vi "New Client.vi"(8 "error in (no error)":errorcluster, 9 "timeout ms (5000)":i32=5000, 11 "WebSocket URL":string) -> (0 "error out":errorcluster, 3 "WebSocket Client out":refnum<class "WebSocket Client.lvclass">)   [LabVIEW 2013, in "WebSockets.lvlib" / "WebSocket Client.lvclass"]
doc: "Opens a conenction and creates a new WebSocket Client using the NI VISA TCP Socket."
uses:
  WebSocket Client.lvclass
  WebSocket/WebSocket.lvclass/WebSocket.ctl
  WebSocket Client.lvclass/WebSocket Client.ctl
  WebSocket/Write Socket.vi
  Write URL.vi
  Sockets/VISA TCP Socket/VISA TCP.lvclass
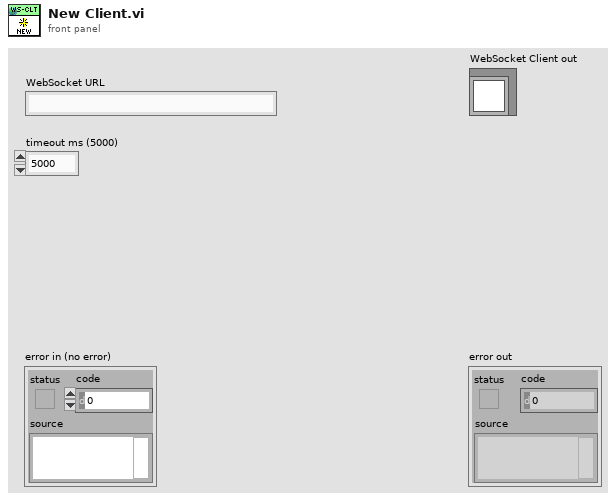
[diagram p1: front panel]
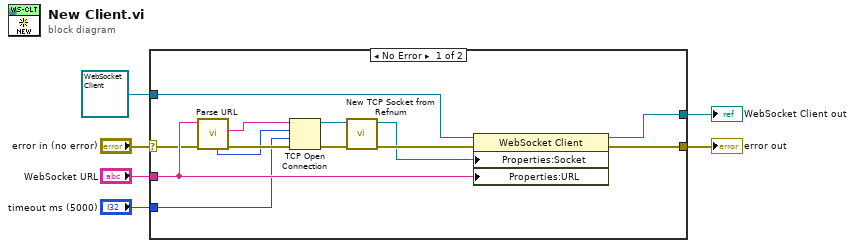
[diagram p0: block diagram]
diagram:
  n1 = case shown="No Error" "error in (no error)" {
    selector: "error in (no error)" -> [w7 w21]
    tunnel: refnum<class "WebSocket Client.lvclass"> refnum ("WebSocket Client in") -> [w19 w20]
    tunnel: [w18 w20] -> w5
    tunnel: [w17 w21] -> w4
    tunnel: "WebSocket URL" -> [w16 _]
    tunnel: "timeout ms (5000)" -> [w9 _]
    frame No Error {
      n2 = call "Parse URL.vi"("error in (no error)"=w7, "WebSocket URL"=w16) -> ("error out"=w10:errorcluster, "host"=w15:string, "port"=w8:u16)  [unwired: 5 in, 2 out]
      n3 = TCP Open Connection(address=w15, remote port or service name=w8, timeout ms (60000)=w9, error in (no error)=w10) -> (connection ID=w13:refnum<k5>, error out=w14:errorcluster)  [unwired: 1 in]
      n4 = call "New TCP Socket from Refnum.vi"("error in (no error)"=w14, "TCP Network Connection Refnum"=w13) -> ("error out"=w12:errorcluster, "VISA TCP out"=w11:refnum<class "VISA TCP.lvclass">)  [unwired: 8 in]
      n5 = property class="WebSocket Client"(reference=w19, error in=w12, "Properties:Socket"=w11, "Properties:URL"=w16) -> (reference out=w18:refnum<class "WebSocket Client.lvclass">, error out=w17:errorcluster)
    }
    frame Error {
    }
  }
  "error out" <- w4
  "WebSocket Client out" <- w5
